vi "Read KeysChanged event.vi"(8 "error in (no error)":errorcluster, 11 "SMO.Configurable in":refnum<class "SMO.Configurable.lvclass">) -> (0 "error out":errorcluster, 2 "keys changed event":refnum<user-event>, 3 "SMO.Configurable out":refnum<class "SMO.Configurable.lvclass">)   [LabVIEW 2013, in "SMO.Configurable.lvclass"]
uses:
  SMO.Configurable.lvclass
  SMO.Configurable.lvclass/SMO.Configurable.ctl
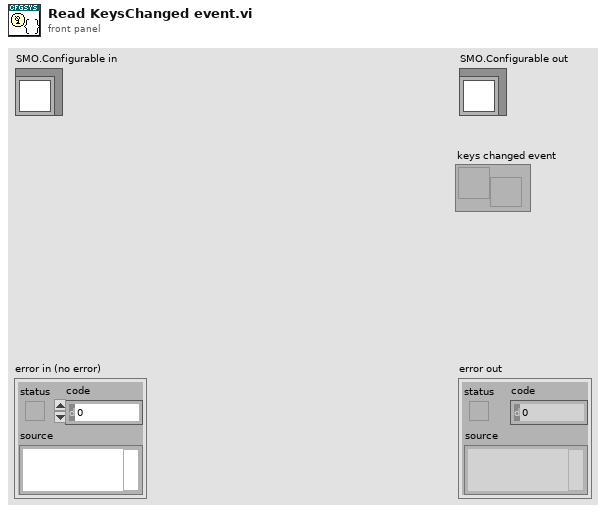
[diagram p1: front panel]
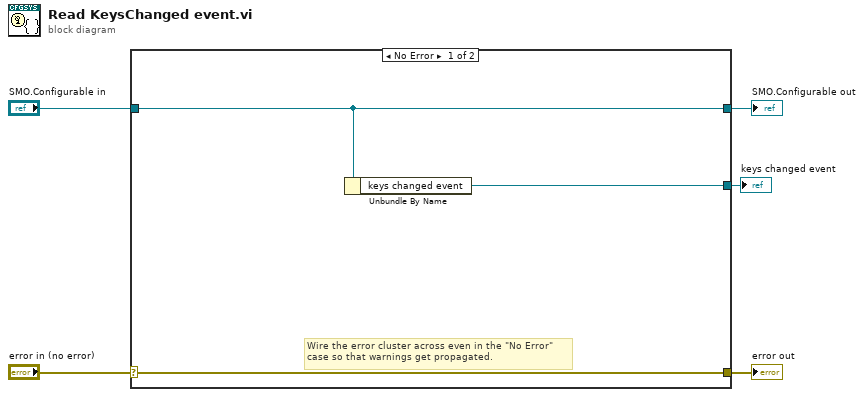
[diagram p0: block diagram]
diagram:
  n1 = case shown="No Error" "error in (no error)" {
    selector: "error in (no error)" -> [w8 w10]
    tunnel: [w8 w10] -> w4
    tunnel: [w7 w9] -> w2
    tunnel: "SMO.Configurable in" -> [w7 w9]
    tunnel: [w6 _] -> w1
    frame No Error {
      # "Wire the error cluster across even in the \"No Error\"\ncase so that warnings get propagated."
      n2 = Unbundle By Name(w7) -> ("keys changed event"=w6:refnum<user-event>)
    }
    frame Error {
    }
  }
  "error out" <- w4
  "SMO.Configurable out" <- w2
  "keys changed event" <- w1
